vi "Disconnect.vi"(8 "error in (no error)":errorcluster, 11 "PXIe5105 in":refnum<class "PXIe5105.lvclass">) -> (0 "error out":errorcluster, 3 "PXIe5105 out":refnum<class "PXIe5105.lvclass">)   [LabVIEW 2018, in "PXIe5105.lvlib" / "PXIe5105.lvclass"]
doc: "This Override method is used finalize the communication session with the Oscope instrument."
uses:
  PXIe5105.lvclass
  PXIe5105.lvclass/PXIe5105.ctl
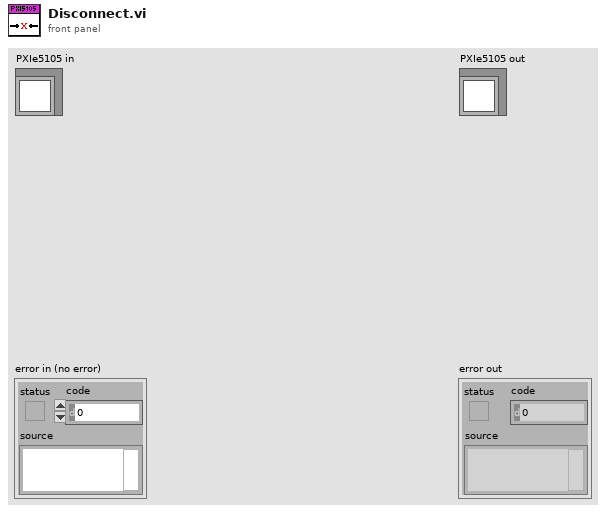
[diagram p1: front panel]
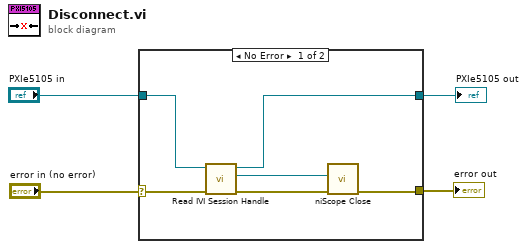
[diagram p0: block diagram]
diagram:
  n1 = case shown="No Error" "error in (no error)" {
    selector: "error in (no error)" -> [w7 w12]
    tunnel: [w10 w12] -> w3
    tunnel: [w8 w11] -> w2
    tunnel: "PXIe5105 in" -> [w9 w11]
    frame No Error {
      n2 = call "Read IVI Session Handle.vi"("error in (no error)"=w7, "PXIe5105 in"=w9) -> ("error out"=w6:errorcluster, "IVI Session Handle"=w5:refnum<k15>, "PXIe5105 out"=w8:refnum<class "PXIe5105.lvclass">)  [unwired: 7 in]
      n3 = call <instrlib>:"niScope Close.vi"("instrument handle"=w5, "error in"=w6) -> ("error out"=w10:errorcluster)  [unwired: 13 in]
    }
    frame Error {
    }
  }
  "error out" <- w3
  "PXIe5105 out" <- w2
